vi "Untitled 1.vi"() -> ()   [LabVIEW 2020]
uses:
  Global 1.vi
panel:
  in  "stop":bool
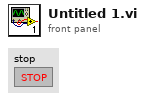
[diagram p1: front panel]
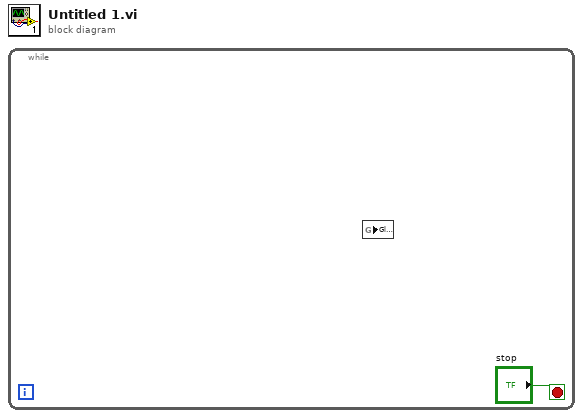
[diagram p0: block diagram]
diagram:
  n1 = while {
    stop <- "stop" stop-if-true
    n2 = global read "Global 1.vi" item#-1() -> ()  [unwired: 1 in]
  }
